vi "Array Edit.vi"(9 "Number of Points":i32, 11 "Y-values":dbl[](array[numeric])) -> (3 "Editted Y Values":dbl[](array[numeric]))   [LabVIEW 2014]
panel:
  # "Array Edit VI"
  # "Outputs"
  # "Inputs"
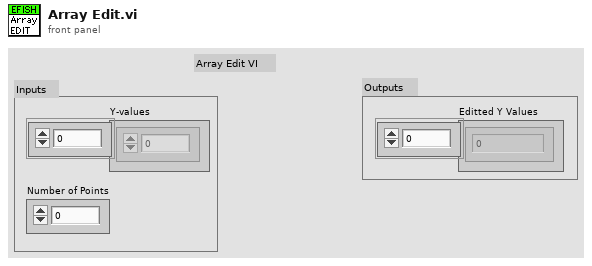
[diagram p1: front panel]
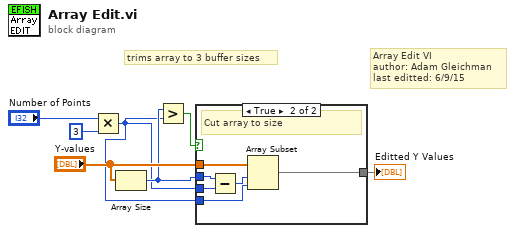
[diagram p0: block diagram]
diagram:
  # "Array Edit VI\nauthor: Adam Gleichman\nlast editted: 6/9/15"
  # "trims array to 3 buffer sizes"
  n1 = Multiply(x="Number of Points", y=3) -> (x*y=w2:i32)
  n2 = Array Size(array="Y-values") -> (size(s)=w5:i32)
  n3 = Greater?(x=w5, y=w2) -> (0:w7:bool)
  n4 = case shown="True" w7 {
    tunnel: "Y-values" -> [w8 w14]
    tunnel: w2 -> [_ w13]
    tunnel: w5 -> [_ w12]
    tunnel: w2 -> [_ w11]
    tunnel: [w8 w9] -> w4
    frame False {
      # "no need to edit"
    }
    frame True {
      # "Cut array to size"
      n5 = Subtract(x=w12, y=w11) -> (x-y=w10:i32)
      n6 = Array Subset(array=w14, index=w10, length=w13) -> (w9:dbl[])
    }
  }
  "Editted Y Values" <- w4
